vi "numero_rand_1_10.vi"() -> ()   [LabVIEW 2020]
panel:
  in  "Numeric":i32
  out "number (0 to 1)":dbl
  out "I":i32
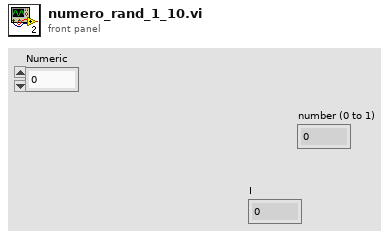
[diagram p1: front panel]
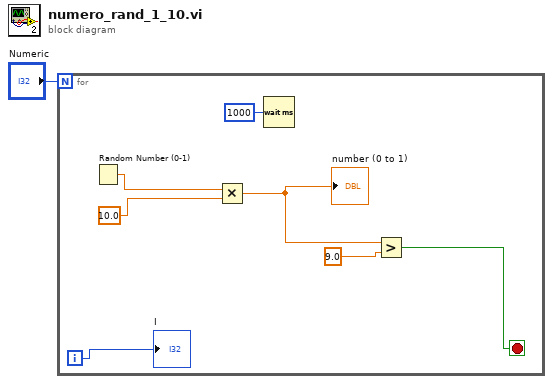
[diagram p0: block diagram]
diagram:
  n1 = for {
    N: "Numeric" -> [_]
    i -> [w6]
    stop <- w2 stop-if-true
    n2 = Random Number (0-1)() -> (number: 0 to 1=w4:dbl)
    n3 = Multiply(x=w4, y=10.0 ("number (0 to 1)")) -> (x*y=w3:dbl)
    "number (0 to 1)" <- w3
    n4 = Wait (ms)(milliseconds to wait=u32 1000) -> ()  [unwired: 1 out]
    n5 = Greater?(x=w3, y=9.0 ("x")) -> (0:w2:bool)
    "I" <- w6
  }
